vi "Set_table_speed.vi"(8 "Z IN":dbl caption="Vitesse Foyer", 9 "Accel IN":dbl caption="Accélération", 10 "Fast IN":dbl caption="Vitesse Rapide", 11 "slow IN":dbl caption="Vitesse Lente") -> (0 "Z OUT":dbl, 1 "Accel OUT":dbl caption="Accélération", 2 "Fast OUT":dbl caption="Vitesse Rapide", 3 "slow OUT":dbl caption="Vitesse Lente")   [LabVIEW 2019]
panel:
  in  "undo":bool
  in  "accept":bool
  # "[pas/sec]"
  # "[pas/sec]"
  # "[pas/sec^2]"
  # "[pas/sec]"
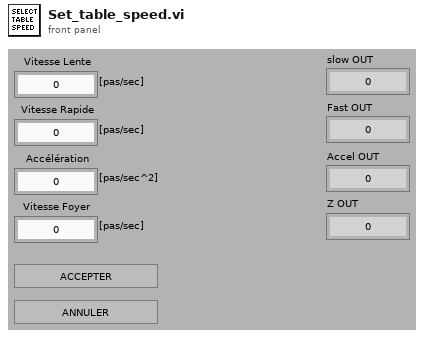
[diagram p1: front panel]
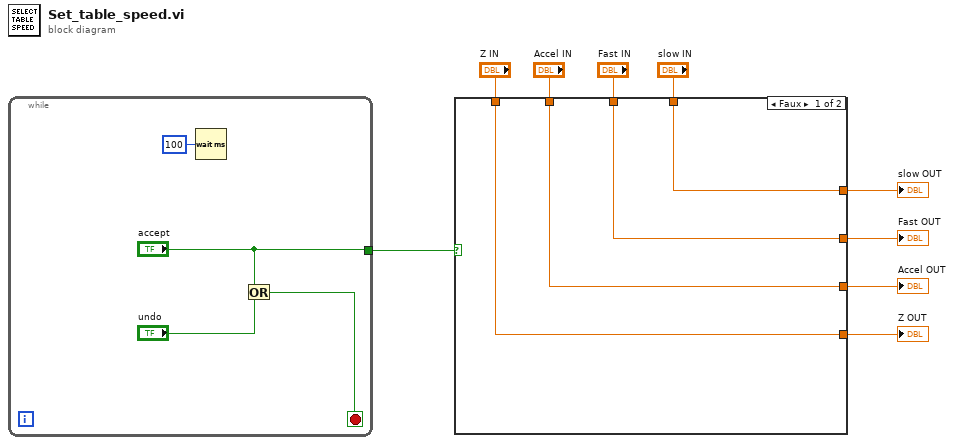
[diagram p0: block diagram]
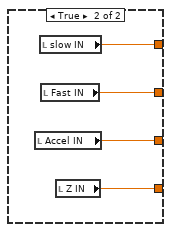
[diagram p2: hidden frame]
diagram:
  n1 = while {
    tunnel: ["accept"] -> w1
    stop <- w11 stop-if-true
    n2 = Wait (ms)(milliseconds to wait=u32 100) -> ()  [unwired: 1 out]
    n3 = Or(x="accept", y="undo") -> (x .or. y?=w11:bool)
  }
  n4 = case shown="Faux" w1 {
    tunnel: [w17 w18] -> w9
    tunnel: [w16 w19] -> w8
    tunnel: [w15 w20] -> w7
    tunnel: [w14 w21] -> w6
    tunnel: "Z IN" -> [w17 _]
    tunnel: "Accel IN" -> [w16 _]
    tunnel: "Fast IN" -> [w15 _]
    tunnel: "slow IN" -> [w14 _]
    frame False {
    }
    frame True {
      n5 = local read "Accel IN"() -> (w19:dbl)
      n6 = local read "slow IN"() -> (w21:dbl)
      n7 = local read "Fast IN"() -> (w20:dbl)
      n8 = local read "Z IN"() -> (w18:dbl)
    }
  }
  "slow OUT" <- w6
  "Fast OUT" <- w7
  "Accel OUT" <- w8
  "Z OUT" <- w9
